vi "rs3 Advanced get Rau Threshold3.vi"(8 "error in (no error)":errorcluster, 10 "mode":i32, 11 "device in":u64) -> (0 "error out 2":errorcluster, 1 "error":u64, 2 "ST Rau Threshold":T1, 3 "Dev out":u64)   [LabVIEW 2017, in "libRealSense3.lvlib"]
doc: "Opens communication to a specific RealSense Device."
uses:
  libRealSense3.lvlib
  realsense2.dll
panel:
  # "RS3 Adv. Get RAU Threshold2"
  # "(C) 2017 Intel Corp.,  AGJ"
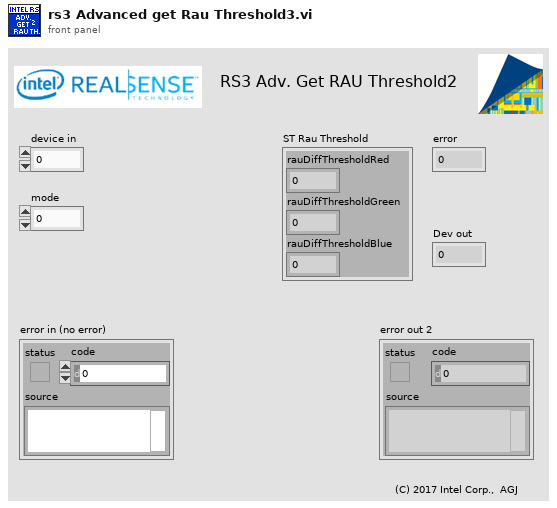
[diagram p1: front panel]
types:
  T1 = cluster{"rauDiffThresholdRed":u32, "rauDiffThresholdGreen":u32, "rauDiffThresholdBlue":u32}
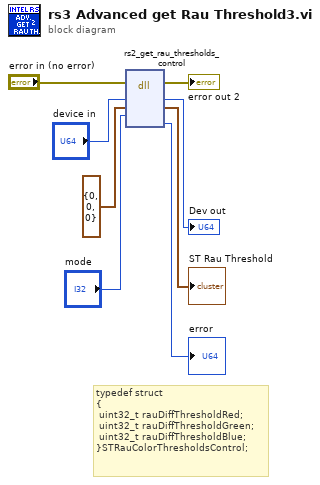
[diagram p0: block diagram]
diagram:
  # "typedef struct\n{\n\tuint32_t rauDiffThresholdRed;\n\tuint32_t rauDiffThresholdGreen;\n\tuint32_t rauDiffThresholdBlue;\n}STRauColorThresholdsControl;"
  n1 = dll-call lib="C:/Users/agrunnet/Documents/libRealSense6/realsense2.dll" fn="rs2_get_rau_thresholds_control"(error in="error in (no error)", "device"="device in", "ST Rau Threshold"=T1 {"rauDiffThresholdRed"=0, "rauDiffThresholdGreen"=0, "rauDiffThresholdBlue"=0} ("output cluster"), "mode"="mode") -> (error out=→"error out 2":errorcluster, "device"=→"Dev out":u64, "ST Rau Threshold"=→"ST Rau Threshold":T1, "error"=→"error":u64)  [unwired: 5 in, 1 out]
